vi "testDifferent.vi"() -> ()   [LabVIEW 2017, in "Assertion.Tests.lvlib" / "AssertNotEquals.lvlib"]
uses:
  AssertNotEquals.lvlib
  1f9a11cc-cfa7-4d0b-86bd-96debd215748.vi
  Constraint/IsEqual/IsEqual.lvclass
  C:/Users/de200256/Code/logmanoriginal/lvunit/Constraint/Constraint/Constraint.lvclass
  Constraint/IsEqual/Create.vi
  Constraint/LogicalNot/LogicalNot.lvclass
  Constraint/UnaryOperator/UnaryOperator.lvclass
  Assertion/Assertion.lvlib
panel:
  out "error out":errorcluster
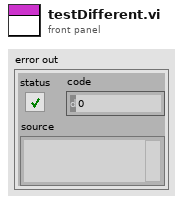
[diagram p1: front panel]
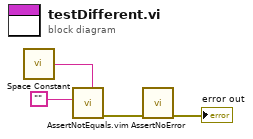
[diagram p0: block diagram]
diagram:
  n1 = call <vilib>:"Space Constant.vi"() -> ("String"=w3:string)
  n2 = call "AssertNotEquals.vim"("Expected"=w3, "Actual"="") -> ("error out"=w2:errorcluster)  [unwired: 9 in]
  n3 = call "AssertNoError.vi"("error in (no error)"=w2) -> ("error out"=→"error out":errorcluster)  [unwired: 10 in]
